vi "lvEtherbone.socket_open.vi"(3 "port":i32, 4 "flags":T2 items=["EB_UDP_MODE", "EB_FEC_MODE"], 5 "error in (no error)":errorcluster) -> (13 "eb_status":T1, 14 "eb_socket_ID":i32, 19 "error out":errorcluster)   [LabVIEW 2009, in "lvEtherbone.lvlib"]
doc: "//-----------------------------------------------------------------------------------\n// author : Dietrich Beck, GSI-Darmstadt\n// purpose : Open an Etherbone socket for communicating with remote devices.\n// The port parameter is optional; 0 lets the operating system choose.\n// The socket_ID must be kept for releasing allocated resources.\n// returns : lveb_status_t\n//-----------------------------------------------------------------------------------\nETHERBONE_API int lveb_socket_open( int port, //port number\n int flags, //flags \n int *eb_socketID //very important socket ID\n );"
uses:
  lvEtherbone.lvlib
  lvEtherbone.eb_flags_t.ctl
  lvEtherbone.lveb_status_t.ctl
  bin/lvEtherbone.dll
panel:
  in  "eb_status_t":T1
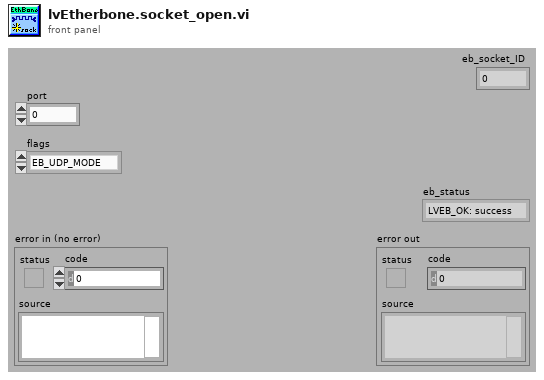
[diagram p1: front panel]
types:
  T1 = typedef "lvEtherbone.lvlib/lvEtherbone.lveb_status_t.ctl" = enum32{"LVEB_OK: success", "LVEB_UNKNOWN: unknown error", "LVEB_OS: operating system forbids access", "LVEB_PORT: port in use or unavailable", "LVEB_ID: ID invalid or out of resources", "LVEB_SOCKET: socket invalid or unavailable", "LVEB_EB: remote address is not Etherbone conformant", "LVEB_IP: bad format or network address", "LVEB_PORTWIDTH: port width error", "LVEB_DEVICEBUSY: Etherbone device still busy", "LVEB_DEVICEFAIL: operation on Wishbone device failed", "LVEB_DEVICEEXIST: Etherbone device already exists, overlaps, or does not exist", "LVEB_TIMEDOUT: a timeout occurred", "LVEB_OVERFLOW: payload of Etherbone exceeded", "LVEB_ADDRESS: bad address", "LVEB_ADDRESSWIDTH: address width error"}
  T2 = typedef "lvEtherbone.lvlib/lvEtherbone.eb_flags_t.ctl" = u32
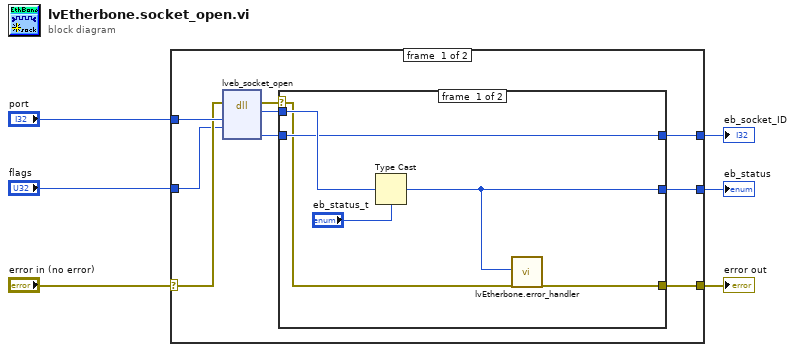
[diagram p0: block diagram]
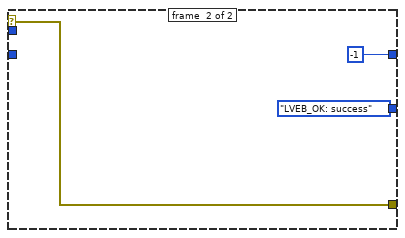
[diagram p2: hidden frame]
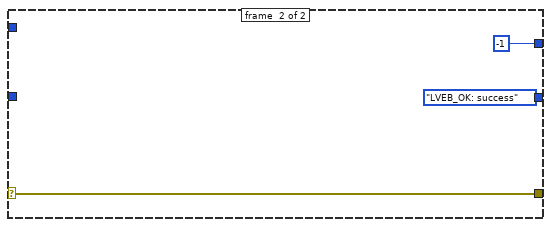
[diagram p3: hidden frame]
diagram:
  n1 = case shown="No Error" "error in (no error)" {
    selector: "error in (no error)" -> [w14 w27]
    tunnel: [w11 w27] -> w5
    tunnel: "port" -> [w15 _]
    tunnel: "flags" -> [w7 _]
    tunnel: [w12 lvEtherbone.lveb_status_t."LVEB_OK: success" ("eb_status_t")] -> w2
    tunnel: [w9 -1 ("eb_socket_ID")] -> w1
    frame #0 {
      n2 = dll-call lib="F:/beck/Project/BEL/SCC/etherbone-core/api/lvEtherbone/bin/lvEtherbone.*" fn="lveb_socket_open"(error in=w14, "port"=w15, "flags"=w7) -> (error out=w8:errorcluster, "eb_status"=w13:i32, "eb_socket_ID"=w10:i32)  [unwired: 5 in, 1 out]
      n3 = case shown="No Error" w8 {
        selector: w8 -> [w16 w24]
        tunnel: w13 -> [w21 _]
        tunnel: [w18 lvEtherbone.lveb_status_t."LVEB_OK: success" ("eb_status_t")] -> w12
        tunnel: [w17 w24] -> w11
        tunnel: w10 -> [w20 _]
        tunnel: [w20 -1 ("eb_socket_ID")] -> w9
        frame #0 {
          n4 = Type Cast(type="eb_status_t", x=w21) -> (*(type *) &x=w18:T1)
          n5 = call "lvEtherbone.error_handler.vi"("eb_status"=w18, "error in"=w16) -> ("error out"=w17:errorcluster)  [unwired: 17 in]
        }
        frame #1 {
        }
      }
    }
    frame #1 {
    }
  }
  "error out" <- w5
  "eb_status" <- w2
  "eb_socket_ID" <- w1
